vi "zad1.vi"() -> ()   [LabVIEW 2025]
uses:
  enum.ctl
  090708c6-a5c4-493d-9c6e-af7f27ae1390.vi
  <vilib>/Array/Sort 2D Array - Pop Stack.vi
  <vilib>/Array/Sort 2D Array - Push Stack.vi
  090708c6-a5c4-493d-9c6e-af7f27ae1390.vi/269d4b3b-47f5-49e3-8884-44851e4dd9d5.vi
  090708c6-a5c4-493d-9c6e-af7f27ae1390.vi/6d99389c-673d-4efb-bf33-19b32bcf4cf8.vi
panel:
  out "Sorted Array":dbl[][](array[numeric])
  in  "Sort by:":T1=enum."Row"
  in  "Select column":i32
  in  "Select row":i32
  in  "Input Array":dbl[][](array[numeric])
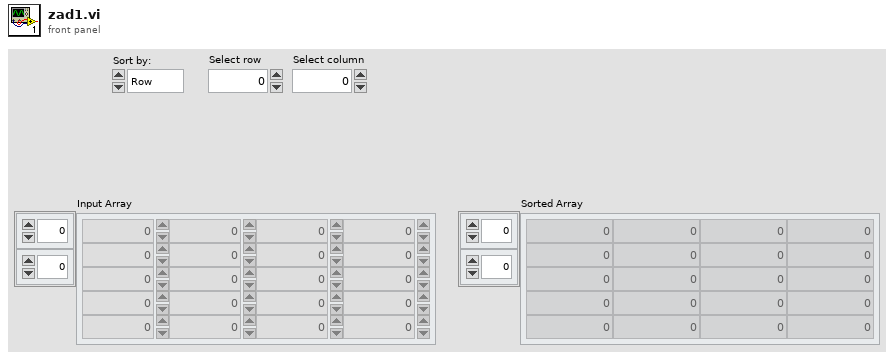
[diagram p1: front panel]
types:
  T1 = typedef "enum.ctl" = enum16{"Column", "Row"}
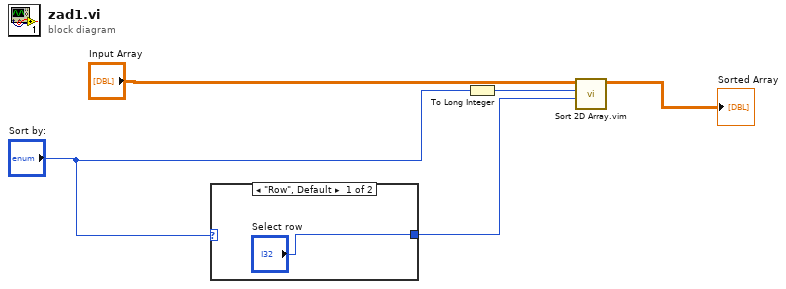
[diagram p0: block diagram]
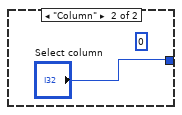
[diagram p2: hidden frame]
diagram:
  n1 = case shown="\"Row\", Default" "Sort by:" {
    tunnel: ["Select row" "Select column"] -> w1
    frame "Row", Default {
    }
    frame "Column" {
      (unwired) 0
    }
  }
  n2 = To Long Integer(number="Sort by:") -> (32bit integer=w3:i32)
  n3 = call "Sort 2D Array.vim"("index"=w1, "dimension to index (column)"=w3, "2D array"="Input Array") -> ("sorted 2D array"=→"Sorted Array":dbl[][])  [unwired: 7 in, 1 out]
